vi "Test Caller.vi"   [LabVIEW 2021, in "Text-Based VI Icon Unit Tests.lvlib"]
doc: "Calls all test related to the Text Based VI Icon.lvlib functions\n\nRegister all functions under this VI to ensure that the test is called in the future."
uses:
  Text-Based VI Icon Unit Tests.lvlib
  <vilib>/addons/_JKI Toolkits/Caraya/classes/Test/Test.lvclass
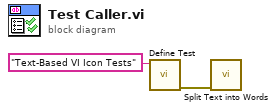
[diagram p0: block diagram]
diagram:
  n1 = call <vilib>:"Define Test.vi"("Label (VI Title)"="Text-Based VI Icon Tests") -> ("error out"=w1:errorcluster)  [unwired: 9 in, 1 out]
  n2 = call "Split Text into Words.vi"("error in (no error)"=w1) -> ()  [unwired: 10 in, 1 out]
